vi "ScanMultChannel_DCV.vi"(7 "VISA resource name":refnum<visa-resource-name>="COM5", 8 "error in (no error)":errorcluster, 9 "Descripbe":string="Start test", 11 "Limit input":string="CH101~CH116") -> (0 "error out":errorcluster={"status"=TRUE, "code"=-1073807343, "source"="Property Node (arg 1) in VISA Configure Serial Port (Instr).vi->ReadChanel.vi->CheckTestStart.vi"}, 1 "TestData":string="0.000000-----0.000000", 2 "TestResult":bool, 3 "Limit out":string="1.2------1.6", 4 "Descripbe output":string="Start test   (CH116)", 5 "Multimeter":refnum<visa-resource-name>="USB0")   [LabVIEW 2013]
uses:
  <vilib>/Utility/error.llb/whitespace.ctl
  MainProgram/Control/Buffer.vi
panel:
  out "testlist":dbl[](array[numeric])
  out "VISA resource name out":refnum<visa-resource-name>="COM5"
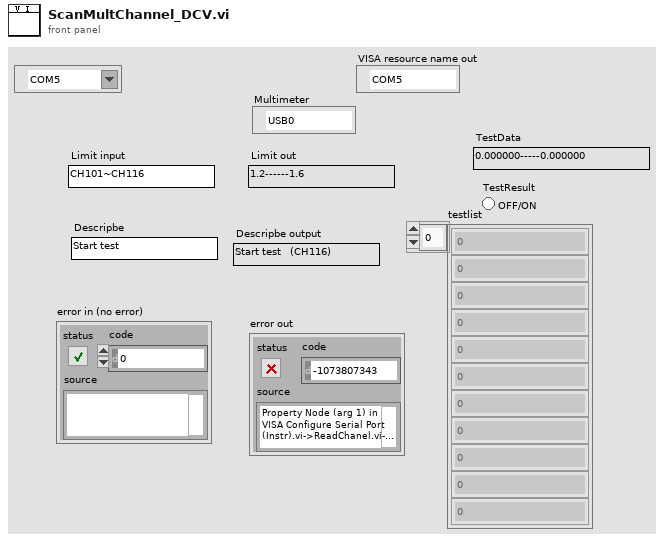
[diagram p1: front panel]
types:
  T1 = typedef "whitespace.ctl" = u16
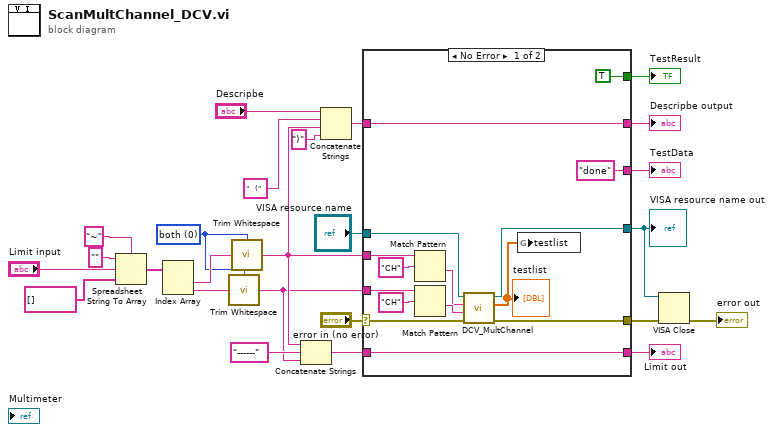
[diagram p0: block diagram]
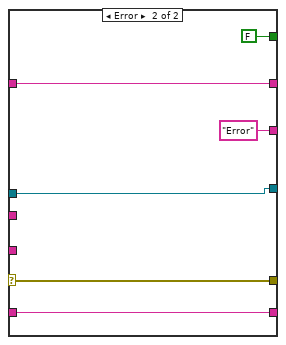
[diagram p2: hidden frame]
diagram:
  w18 = T1 0 items=["both", "start of string", "end of string"] ("location (both)")
  n1 = Spreadsheet String To Array(delimiter (Tab)="~", format string="", spreadsheet string="Limit input", array type (2D Dbl)=string[] []) -> (array=w21:string[])
  n2 = Index Array(array=w21) -> (element #1=w20:string, element #2=w19:string)  [unwired: 2 in]
  n3 = call <vilib>:"Trim Whitespace.vi"("string"=w19, "location (both)"=w18) -> ("trimmed string"=w1:string)
  n4 = call <vilib>:"Trim Whitespace.vi"("string"=w20, "location (both)"=w18) -> ("trimmed string"=w2:string)
  n5 = Concatenate Strings(w2, "------" ("string"), w1) -> (w13:string)
  n6 = Concatenate Strings("Descripbe", "   (" ("string"), w2, ")" ("string")) -> (w8:string)
  n7 = case shown="No Error" "error in (no error)" {
    selector: "error in (no error)" -> [w36 w46]
    tunnel: [w35 w46] -> w6
    tunnel: w2 -> [w38 _]
    tunnel: [TRUE FALSE] -> w17
    tunnel: [w39 w44] -> w14
    tunnel: w13 -> [w39 w44]
    tunnel: [w37 w43] -> w12
    tunnel: w8 -> [w37 w43]
    tunnel: ["done" ("read buffer") "Error" ("read buffer")] -> w7
    tunnel: "VISA resource name" -> [w34 w41]
    tunnel: [w33 w41] -> w3
    tunnel: w1 -> [w28 _]
    frame No Error {
      n8 = Match Pattern(string=w38, regular expression="CH") -> (after substring=w26:string)  [unwired: 1 in, 3 out]
      n9 = Match Pattern(string=w28, regular expression="CH") -> (after substring=w27:string)  [unwired: 1 in, 3 out]
      n10 = call "DCV_MultChannel.vi"("Error In"=w36, "End channel"=w27, "Start channel"=w26, "VISA resource name"=w34) -> ("Error Out"=w35:errorcluster, "testlist"=w30:dbl[], "VISA resource name out"=w33:refnum<visa-resource-name>)  [unwired: 5 in]
      "testlist" <- w30
      n11 = global write "Buffer.vi" "testlist"(w30) -> ()
    }
    frame Error {
    }
  }
  "TestResult" <- w17
  "TestData" <- w7
  "Limit out" <- w14
  "Descripbe output" <- w12
  "VISA resource name out" <- w3
  n12 = VISA Close(VISA resource name=w3, error in (no error)=w6) -> (error out=→"error out":errorcluster)
